vi "Gui_SetupExcitation.vi"(7 "Variant For Path":variant, 8 "error in (no error)":errorcluster, 11 "Variant":variant) -> (0 "error out":errorcluster caption="sortie d'erreur", 3 "Variant Output":variant)   [LabVIEW 2017]
uses:
  controls/SEQUENCE_Inputs.ctl
  controls/TRAPPING_Inputs.ctl
  controls/EXCIT_Inputs.ctl
  controls/DATA_Inputs.ctl
  controls/TIMING_Inputs.ctl
  controls/PROCESSING_Inputs.ctl
  controls/EXPERT_Inputs.ctl
  controls/DIGIT_5122_Inputs.ctl
  <instrlib>/niScope/Controls/niScope trigger source.ctl
  controls/HSDIO_6541_Inputs.ctl
  <instrlib>/niHSDIO/niHSDIO.llb/niHSDIO_ctl Trigger Source Values (Ring).ctl
  controls/SOFTWARE_Inputs.ctl
  controls/AO_6711_Inputs.ctl
  controls/AWG_5421_Inputs.ctl
  <instrlib>/niFgen/niFgen.llb/niFgen_ctl Trigger Source Values (Ring).ctl
  controls/XML_Inputs.ctl
  controls/EXCIT_Waveforms_Inputs.ctl
panel:
  in  "SEQUENCE Inputs":T1={"TRAPPING Inputs"={"Number of Channels"=4, "Init Values"=[2.0, 5.0, 5.0, 2.0], "Opening Values"=[0.0, 0.0, 0.0, 0.0], "Trapping Values"=[2.0, 5.0, 5.0, 2.0], "Emptying Values"=[-5.0, -5.0, -5.0, -5.0], "Adiabatic ON"=FALSE, "Adiabatic Duration"=0, "Adiabatic Waveforms"=["Adiabatic_None_2_2_2000.bin", "Adiabatic_Ramp_5_0_2000.bin", "Adiabatic_DoubleRamp_5_0_2000.bin", "Adiabatic_RC_2_0_2000.bin"]}, "EXCIT Inputs"={"Number of Excitations"=1, "Script Text"="", "Table of Waveforms"=[]}, "DATA Inputs"={"Record Length"=8192, "Sample Rate"=4.0, "Data Type"=0, "Vertical Range"=0.0, "Acquisition Duration"=100000.0}, "TIMING Inputs"={"Number of Acquisitions "=1, "Number of Accumulations"=1, "Table of Waveforms"=[], "Script Text"=""}, "PROCESSING  Inputs"={"Reference Mass"=300.0939, "Cyclotron Freq"=255.727, "Magnetron Freq"=0.001}} {"PROCESSING  Inputs"."Magnetron Freq" format="%.5g"; "PROCESSING  Inputs"."Cyclotron Freq" format="%.5g"; "PROCESSING  Inputs"."Reference Mass" format="%.5g"; "TIMING Inputs"."Number of Accumulations" min=0 max=50 step=1; "TIMING Inputs"."Number of Acquisitions" min=1 max=10 step=1; "DATA Inputs"."Vertical Range" items=["0.2"=0.2, "0.4"=0.4, "1"=1.0, "2"=2.0, "4"=4.0, "10"=10.0]; "DATA Inputs"."Data Type" items=["I16", "DBL"]; "DATA Inputs"."Sample Rate" items=["1 MHz"=1000000.0, "2 MHz"=2000000.0, "5 MHz"=5000000.0, "10 MHz"=10000000.0, "20 MHz"=20000000.0, "25 MHz"=25000000.0, "50 MHz"=50000000.0, "100 MHz"=100000000.0]; "EXCIT Inputs"."Number of Excitations" min=1 max=10; "TRAPPING Inputs"."Trapping Values" min=-10.0 max=10.0; "TRAPPING Inputs"."Init Values" min=-10.0 max=10.0; "TRAPPING Inputs"."Emptying Values" min=-10.0 max=10.0; "TRAPPING Inputs"."Opening Values" min=-10.0 max=10.0}
  out "Script File":string
  out "Script text":string
  out "Table of Waveforms":string[](array[string])
  in  "EXCIT 5":bool
  in  "EXCIT 4":bool
  in  "EXCIT 3":bool
  in  "EXCIT 2":bool
  in  "EXCIT 1":bool
  in  "Number of excitations":i32 min=0 max=5 step=1
  in  "OK":bool
  # "GO_out"
  # "Gout"
  # "GI_in"
  # "Gin"
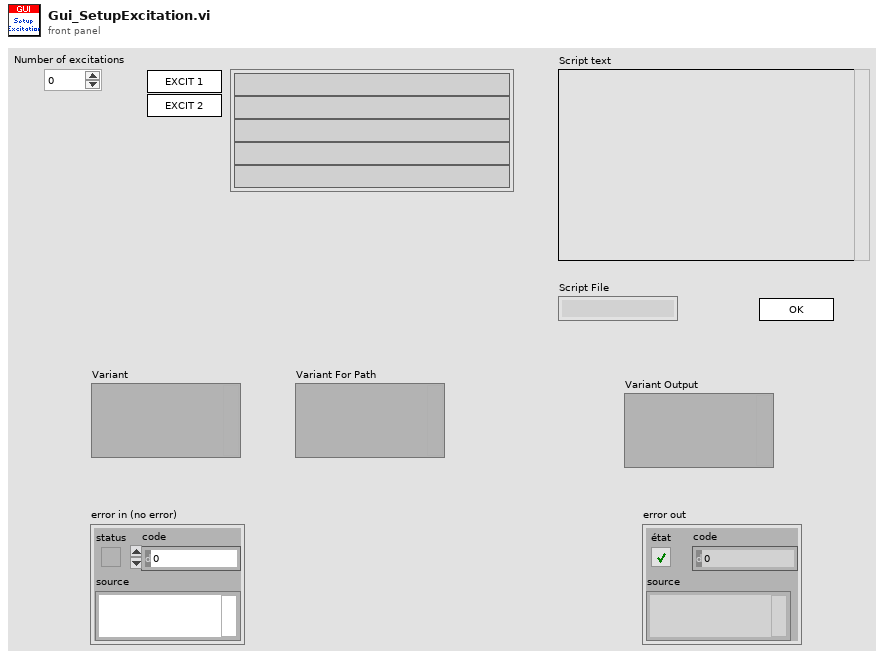
[diagram p1: front panel]
types:
  T1 = typedef "SEQUENCE_Inputs.ctl" = cluster{"TRAPPING Inputs":T2, "EXCIT Inputs":T3, "DATA Inputs":T4, "TIMING Inputs":T5, "PROCESSING  Inputs":T6}
  T2 = typedef "TRAPPING_Inputs.ctl" = cluster{"Number of Channels":i32, "Init Values":dbl[], "Opening Values":dbl[], "Trapping Values":dbl[], "Emptying Values":dbl[], "Adiabatic ON":bool, "Adiabatic Duration":i32, "Adiabatic Waveforms":string[]}
  T3 = typedef "EXCIT_Inputs.ctl" = cluster{"Number of Excitations":i32, "Script Text":string, "Table of Waveforms":string[]}
  T4 = typedef "DATA_Inputs.ctl" = cluster{"Record Length":i32, "Sample Rate":dbl, "Data Type":u8, "Vertical Range":dbl, "Acquisition Duration":dbl}
  T5 = typedef "TIMING_Inputs.ctl" = cluster{"Number of Acquisitions ":i16, "Number of Accumulations":i16, "Table of Waveforms":string[], "Script Text":string}
  T6 = typedef "PROCESSING_Inputs.ctl" = cluster{"Reference Mass":dbl, "Cyclotron Freq":dbl, "Magnetron Freq":dbl}
  T7 = typedef "EXCIT_Waveforms_Inputs.ctl" = cluster{"Excit Form":enum16{"Sinus", "Chirp", "Swift", "TwoSwift", "Ramp"}, "Amplitude":dbl, "Start Frequency":dbl, "End Frequency":dbl, "Duration":dbl, "Sampling Frequency":dbl, "Swift Factor":dbl, "Chirp Apodisation":dbl, "Amplitude 2":dbl, "Start Frequency 2":dbl, "End Frequency 2":dbl}
  T8 = typedef "EXPERT_Inputs.ctl" = cluster{"DIGIT 5122 Inputs":T9, "HSDIO 6541 Inputs":T11, "SOFTWARE Inputs":T13, "AO 6711 Inputs":T14, "AWG 5421 Inputs":T15, "XML Inputs":T17}
  T9 = typedef "DIGIT_5122_Inputs.ctl" = cluster{"Sample Rate":dbl, "Resource Name":refnum<k15>, "Channel Name":string, "Trigger Source":T10, "Vertical Range":dbl, "Trigger Level":dbl}
  T10 = typedef "niScope trigger source.ctl" = string
  T11 = typedef "HSDIO_6541_Inputs.ctl" = cluster{"Resource Name":refnum<k15>, "Clock Rate":dbl, "Trigger Source":T12}
  T12 = typedef "niHSDIO_ctl Trigger Source Values (Ring).ctl" = string
  T13 = typedef "SOFTWARE_Inputs.ctl" = cluster{"Application Directory":path, "Software Version":string, "Data Path":path, "XML Path":path, "XML File Filter":string, "XML Saved Path":path, "Excit Scripts Path":path, "Excit Scripts File Filter":string, "Excit Waveforms Path":path, "Excit Waveforms File Filter":string, "Timing Scripts Path":path, "Timing Scripts File Filter":string, "Timing Waveforms Path":path, "Timing Waveforms File Filter":string, "Trapping Waveforms Path":path, "Trapping Waveforms File Filter":string}
  T14 = typedef "AO_6711_Inputs.ctl" = cluster{"Physical Channels":tag, "Min Voltage":dbl, "Max Voltage":dbl, "Trigger Source":tag, "Counter":tag}
  T15 = typedef "AWG_5421_Inputs.ctl" = cluster{"Resource Name":refnum<k15>, "Sample Rate":dbl, "Trigger Type":u16, "Trigger Source":T16, "Waveform Gain":dbl, "Digital Filter ON":bool}
  T16 = typedef "niFgen_ctl Trigger Source Values (Ring).ctl" = string
  T17 = typedef "XML_Inputs.ctl" = cluster{"Version Tag Name":string, "Version String":string}
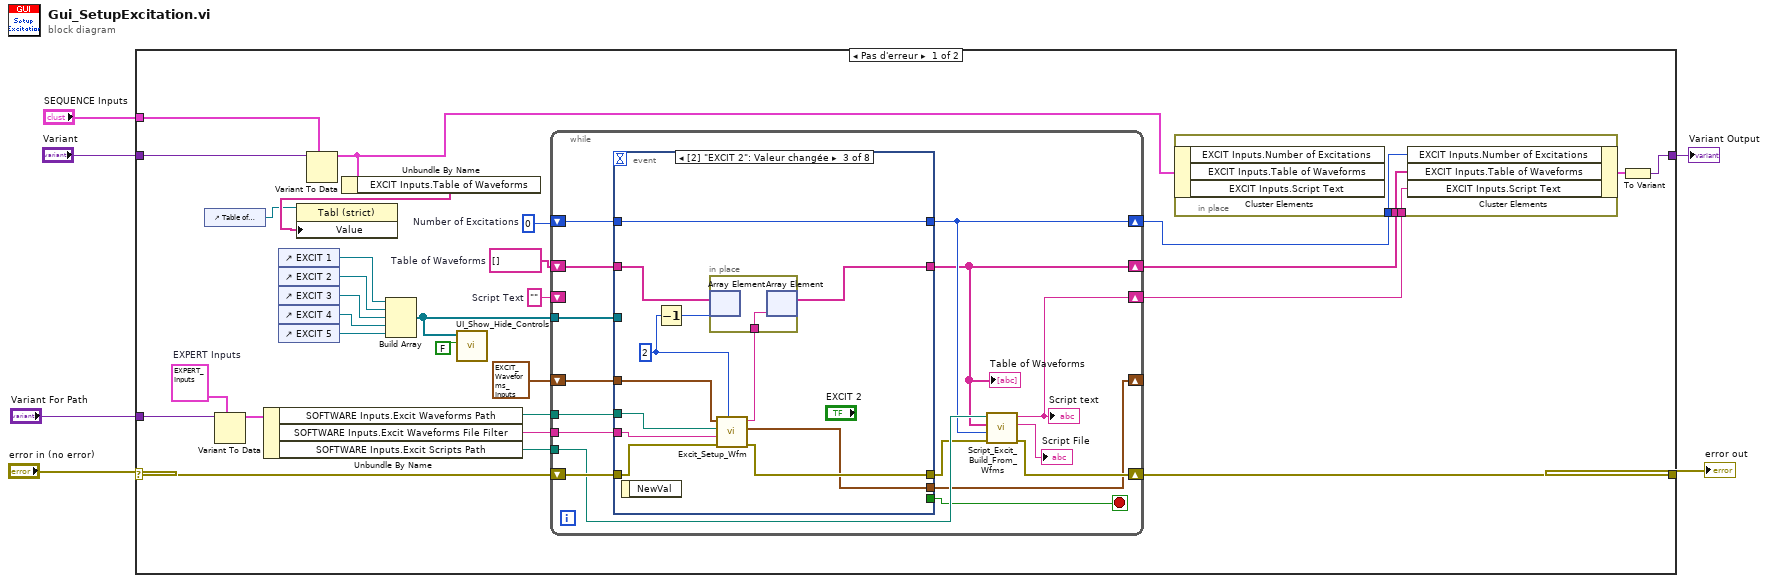
[diagram p0: block diagram]
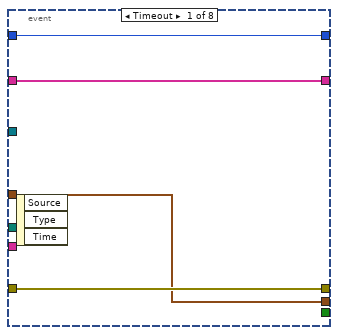
[diagram p2: hidden frame]
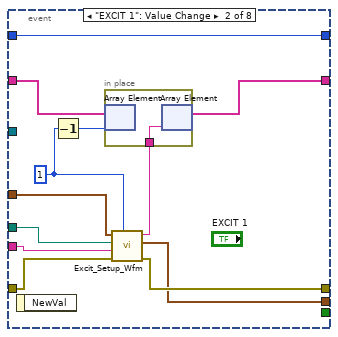
[diagram p3: hidden frame]
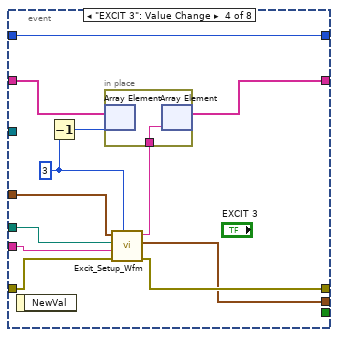
[diagram p4: hidden frame]
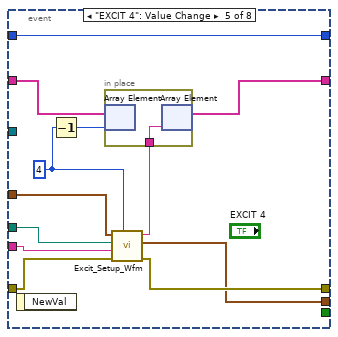
[diagram p5: hidden frame]
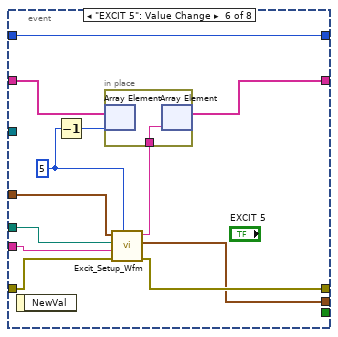
[diagram p6: hidden frame]
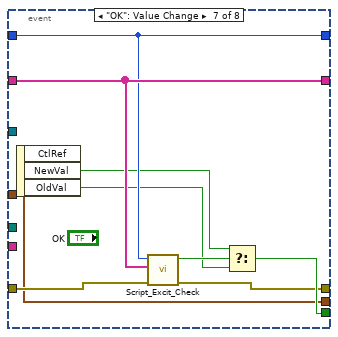
[diagram p7: hidden frame]
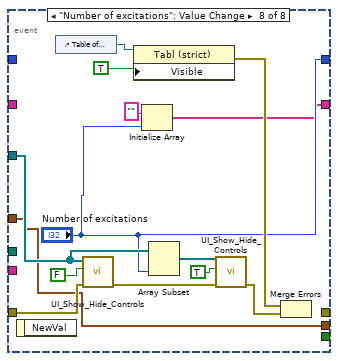
[diagram p8: hidden frame]
diagram:
  n1 = case shown="Pas d'erreur" "error in (no error)" {
    selector: "error in (no error)" -> [w35 w148]
    tunnel: [w27 w148] -> w5
    tunnel: "Variant" -> [w17 w147]
    tunnel: "Variant For Path" -> [w23 _]
    tunnel: [w12 w147] -> w2
    tunnel: "SEQUENCE Inputs" -> [w7 _]
    frame No Error {
      w18 = ""  # Script Text
      w22 = string[] []  # Table of Waveforms
      w25 = T8 {"DIGIT 5122 Inputs"={"Sample Rate"=1.0, "Resource Name"="Digitizer", "Channel Name"="0", "Trigger Source"="VAL_EXTERNAL", "Vertical Range"=10.0, "Trigger Level"=3.0}, "HSDIO 6541 Inputs"={"Resource Name"="SequencerHSDIO", "Clock Rate"=1000000.0, "Trigger Source"="PFI0"}, "SOFTWARE Inputs"={"Application Directory"=path "D:/S.O.F.T.S/LABVIEW/PIL", "Software Version"="1.0.0", "Data Path"=path "D:/PIRENEA/DATA", "XML Path"=path "D:/PIRENEA/DATA", "XML File Filter"="*.xml", "XML Saved Path"=path "D:/PIRENEA/DATA", "Excit Scripts Path"=path "D:/PIRENEA/EXCIT_SCRIPTS", "Excit Scripts File Filter"="*.txt", "Excit Waveforms Path"=path "D:/PIRENEA/EXCIT_WFMS", "Excit Waveforms File Filter"="*.bin", "Timing Scripts Path"=path "D:/PIRENEA/SEQUENCE_SCRIPTS", "Timing Scripts File Filter"="*.txt", "Timing Waveforms Path"=path "D:/PIRENEA/SEQUENCE_WFMS", "Timing Waveforms File Filter"="*.bin", "Trapping Waveforms Path"=path "D:/PIRENEA/TRAPPING_WFMS", "Trapping Waveforms File Filter"="*.bin"}, "AO 6711 Inputs"={"Physical Channels"="AnalogOutput/ao0:3", "Min Voltage"=-10.0, "Max Voltage"=10.0, "Trigger Source"="/AnalogOutput/PFI0", "Counter"="AnalogOutput/ctr0"}, "AWG 5421 Inputs"={"Resource Name"="WaveformGenerator", "Sample Rate"=0.0, "Trigger Type"=4, "Trigger Source"="PFI0", "Waveform Gain"=0.31, "Digital Filter ON"=TRUE}, "XML Inputs"={"Version Tag Name"="XML_Version", "Version String"="1.0"}}  # EXPERT Inputs
      w26 = 0  # Number of Excitations
      n2 = control-ref of="Table of Waveforms"() -> (w8:refnum<vi>)
      n3 = Variant To Data(type=w25, Variant=w23) -> (data=w24:T8)  [unwired: 1 in, 1 out]
      n4 = Unbundle By Name(w24) -> ("SOFTWARE Inputs.Excit Waveforms Path"=w21:path, "SOFTWARE Inputs.Excit Waveforms File Filter"=w20:string, "SOFTWARE Inputs.Excit Scripts Path"=w19:path)
      n5 = control-ref of="EXCIT 1"() -> (w30:refnum<vi>)
      n6 = control-ref of="EXCIT 2"() -> (w29:refnum<vi>)
      n7 = control-ref of="EXCIT 3"() -> (w31:refnum<vi>)
      n8 = control-ref of="EXCIT 4"() -> (w32:refnum<vi>)
      n9 = control-ref of="EXCIT 5"() -> (w33:refnum<vi>)
      n10 = Variant To Data(type=w7, Variant=w17) -> (data=w10:T1)  [unwired: 1 in, 1 out]
      n11 = Unbundle By Name(w10) -> ("EXCIT Inputs.Table of Waveforms"=w9:string[])
      n12 = property class="Tabl (strict)"(reference=w8, "Value"=w9) -> ()  [unwired: 1 in, 2 out]
      n13 = Build Array(w30, w29, w31, w32, w33) -> (w28:refnum<vi>[])
      n14 = call "UI_Show_Hide_Controls.vi"("Enable ?"=FALSE, "Controls"=w28) -> ()  [unwired: 9 in, 1 out]
      n15 = while {
        shift-right: [w45] -> w27
        shift-left: w35 -> [w54]
        tunnel: w28 -> [w51]
        shift-right: [w47] -> w14
        shift-left: w26 -> [w53]
        shift-right: [w42] -> w16
        shift-left: w22 -> [w52]
        tunnel: w21 -> [w50]
        tunnel: w20 -> [w49]
        tunnel: w19 -> [w48]
        shift-right: [w43] -> w15
        shift-left: w18 -> [_]
        shift-right: [w39] -> _
        shift-left: T7 {"Excit Form"=enum."Sinus", "Amplitude"=100.0, "Start Frequency"=250.0, "End Frequency"=350.0, "Duration"=800.0, "Sampling Frequency"=10.0, "Swift Factor"=0.5, "Chirp Apodisation"=3.5, "Amplitude 2"=100.0, "Start Frequency 2"=250.0, "End Frequency 2"=350.0} ("EXCIT Waveforms Inputs") -> [w40]
        stop <- w41 stop-if-true
        n16 = event shown="[2] \"EXCIT 2\": Valeur changée" {
          selector: _ -> [_ _ _ _ _ _ _ _]
          dyn-events: _ -> [_ _ _ _ _ _ _ _]
          timeout: _ -> [_ _ _ _ _ _ _ _]
          tunnel: w54 -> [w57 w70 w83 w96 w109 w122 w130 w143]
          tunnel: [w57 w69 w82 w95 w108 w121 w125 _] -> w46
          tunnel: w51 -> [_ _ _ _ _ _ _ w140]
          tunnel: w53 -> [w58 w63 w76 w89 w102 w115 w131 _]
          tunnel: [w58 w63 w76 w89 w102 w115 w131 "Number of excitations"] -> w47
          tunnel: w52 -> [w56 w67 w80 w93 w106 w119 w132 _]
          tunnel: [w56 w66 w79 w92 w105 w118 w132 w133] -> w42
          tunnel: w50 -> [_ w65 w78 w91 w104 w117 _ _]
          tunnel: w49 -> [_ w64 w77 w90 w103 w116 _ _]
          tunnel: [_ _ _ _ _ _ w127 _] -> w41
          tunnel: w40 -> [w55 w62 w75 w88 w101 w114 w124 w135]
          tunnel: [w55 w61 w74 w87 w100 w113 w124 w135] -> w39
          event Timeout {
            n17 = event-data() -> ()  [unwired: 1 in, 3 out]
          }
          event "EXCIT 1": Value Change {
            w60 = 1 ("Excit Number")
            n18 = event-data() -> ()  [unwired: 1 in, 1 out]
            n19 = Decrement(x=w60) -> (x-1=w59:i32)
            n20 = call "Excit_Setup_Wfm.vi"("Excit Number"=w60, "error in"=w70, "Excit Waveforms File Filter"=w64, "Excit Waveforms Path"=w65, "EXCIT Waveforms Inputs"=w62) -> ("error out"=w69:errorcluster, "EXCIT Waveforms Inputs"=w61:T7, "Waveform Name"=w68:string)  [unwired: 4 in]
            n21 = in-place {
              in-place-border: w68 -> [w71]
              n22 = in-place-array #1(w67, w59) -> ()  [unwired: 1 out]
              n23 = in-place-array #1(w71) -> (w66:string[])  [unwired: 1 out]
            }
          }
          event "EXCIT 2": Value Change {
            w73 = 2 ("Excit Number")
            n24 = event-data() -> ()  [unwired: 1 in, 1 out]
            n25 = Decrement(x=w73) -> (x-1=w72:i32)
            n26 = call "Excit_Setup_Wfm.vi"("Excit Number"=w73, "error in"=w83, "Excit Waveforms File Filter"=w77, "Excit Waveforms Path"=w78, "EXCIT Waveforms Inputs"=w75) -> ("error out"=w82:errorcluster, "EXCIT Waveforms Inputs"=w74:T7, "Waveform Name"=w81:string)  [unwired: 4 in]
            n27 = in-place {
              in-place-border: w81 -> [w84]
              n28 = in-place-array #2(w80, w72) -> ()  [unwired: 1 out]
              n29 = in-place-array #2(w84) -> (w79:string[])  [unwired: 1 out]
            }
          }
          event "EXCIT 3": Value Change {
            w86 = 3 ("Excit Number")
            n30 = event-data() -> ()  [unwired: 1 in, 1 out]
            n31 = Decrement(x=w86) -> (x-1=w85:i32)
            n32 = call "Excit_Setup_Wfm.vi"("Excit Number"=w86, "error in"=w96, "Excit Waveforms File Filter"=w90, "Excit Waveforms Path"=w91, "EXCIT Waveforms Inputs"=w88) -> ("error out"=w95:errorcluster, "EXCIT Waveforms Inputs"=w87:T7, "Waveform Name"=w94:string)  [unwired: 4 in]
            n33 = in-place {
              in-place-border: w94 -> [w97]
              n34 = in-place-array #3(w93, w85) -> ()  [unwired: 1 out]
              n35 = in-place-array #3(w97) -> (w92:string[])  [unwired: 1 out]
            }
          }
          event "EXCIT 4": Value Change {
            w99 = 4 ("Excit Number")
            n36 = event-data() -> ()  [unwired: 1 in, 1 out]
            n37 = Decrement(x=w99) -> (x-1=w98:i32)
            n38 = call "Excit_Setup_Wfm.vi"("Excit Number"=w99, "error in"=w109, "Excit Waveforms File Filter"=w103, "Excit Waveforms Path"=w104, "EXCIT Waveforms Inputs"=w101) -> ("error out"=w108:errorcluster, "EXCIT Waveforms Inputs"=w100:T7, "Waveform Name"=w107:string)  [unwired: 4 in]
            n39 = in-place {
              in-place-border: w107 -> [w110]
              n40 = in-place-array #4(w106, w98) -> ()  [unwired: 1 out]
              n41 = in-place-array #4(w110) -> (w105:string[])  [unwired: 1 out]
            }
          }
          event "EXCIT 5": Value Change {
            w112 = 5 ("Excit Number")
            n42 = event-data() -> ()  [unwired: 1 in, 1 out]
            n43 = Decrement(x=w112) -> (x-1=w111:i32)
            n44 = call "Excit_Setup_Wfm.vi"("Excit Number"=w112, "error in"=w122, "Excit Waveforms File Filter"=w116, "Excit Waveforms Path"=w117, "EXCIT Waveforms Inputs"=w114) -> ("error out"=w121:errorcluster, "EXCIT Waveforms Inputs"=w113:T7, "Waveform Name"=w120:string)  [unwired: 4 in]
            n45 = in-place {
              in-place-border: w120 -> [w123]
              n46 = in-place-array #5(w119, w111) -> ()  [unwired: 1 out]
              n47 = in-place-array #5(w123) -> (w118:string[])  [unwired: 1 out]
            }
          }
          event "OK": Value Change {
            n48 = event-data() -> ("NewVal"=w126:bool, "OldVal"=w128:bool)  [unwired: 1 in, 1 out]
            n49 = call "Script_Excit_Check.vi"("error in (no error)"=w130, "Table of Waveforms"=w132, "Number of excitations"=w131) -> ("error out"=w125:errorcluster, "Check Result"=w129:bool)  [unwired: 7 in]
            n50 = Select(t=w126, s=w129, f=w128) -> (s? t:f=w127:bool)
          }
          event "Number of excitations": Value Change {
            n51 = event-data() -> ()  [unwired: 1 in, 1 out]
            n52 = control-ref of="Table of Waveforms"() -> (w139:refnum<vi>)
            n53 = call "UI_Show_Hide_Controls.vi"("error in (no error)"=w143, "Enable ?"=FALSE, "Controls"=w140) -> ("error out"=w142:errorcluster)  [unwired: 8 in]
            n54 = property class="Tabl (strict)"(reference=w139, "Visible"=TRUE) -> (error out=w138:errorcluster)  [unwired: 1 in, 1 out]
            n55 = Initialize Array("", "Number of excitations") -> (w133:string[])
            n56 = Array Subset(array=w140, length="Number of excitations") -> (w141:refnum<vi>[])  [unwired: 1 in]
            n57 = call "UI_Show_Hide_Controls.vi"("error in (no error)"=w142, "Enable ?"=TRUE, "Controls"=w141) -> ("error out"=w137:errorcluster)  [unwired: 8 in]
            n58 = Merge Errors(w138, w137) -> ()  [unwired: 1 out]
          }
        }
        "Table of Waveforms" <- w42
        n59 = call "Script_Excit_Build_From_Wfms.vi"("error in (no error)"=w46, "Number of excitations"=w47, "Table of Waveforms"=w42, "Script Path"=w48) -> ("error out"=w45:errorcluster, "Script File"=→"Script File":string, "Script Text"=w43:string)  [unwired: 5 in]
        "Script text" <- w43
      }
      n60 = in-place {
        in-place-border: w14 -> [w38]
        in-place-border: w16 -> [w37]
        in-place-border: w15 -> [w36]
        n61 = in-place-cluster #6(w10) -> ()  [unwired: 3 out]
        n62 = in-place-cluster #6("EXCIT Inputs.Number of Excitations"=w38, "EXCIT Inputs.Table of Waveforms"=w37, "EXCIT Inputs.Script Text"=w36) -> (w13:T1)
      }
      n63 = To Variant(anything=w13) -> (Variant=w12:variant)
    }
    frame Error {
    }
  }
  "error out" <- w5
  "Variant Output" <- w2
